vi "Configure Mask Test.vi"(0 "VISA resource name":refnum<visa-resource-name>, 1 "Enable Mask Test (T: Enable)":bool=TRUE, 5 "Mask Test Source (1: Channel 1)":i32(ring)=1 items=["Channel 1"=1, "Channel 2"=2, "Channel 3"=3, "Channel 4"=4, "Function 1"=5, "Function 2"=6, "Function 3"=7, "Function 4"=8, "Differential 1"=61, "Differential 2"=62, "Common 1"=71, "Common 2"=72, "Equalized"=18], 7 "Mask Trigger Source (1: Channel 1)":i32(ring)=1 items=["Channel 1"=1, "Channel 2"=2, "Channel 3"=3, "Channel 4"=4], 9 "Impedance (0: None)":i32(ring) items=["None", "IMP75", "IMP100", "IMP110", "IMP120"], 11 "error in (no error)":errorcluster, 12 "Run":T2={"Enable Stop on Fail (F: Disable)"=FALSE, "Run Mode (0: Forever)"=0, "Waveform Count (1000)"=1000, "Time (1.0 min)"=1.0} {"Time (1.0 min)" format="%#.1g"; "Run Mode (0: Forever)" items=["Forever", "Waveform", "Time"]}, 13 "Test Options":T3={"Enable Averaging (F: Disable)"=FALSE, "Average Count (16)"=16, "Enable Use File Setup (T: Enable)"=TRUE}, 14 "Pulse Amplitude":T1={"Maximum Amplitude (1 V)"=1.0, "Minimum Amplitude (1 V)"=1.0}) -> (4 "VISA resource name out":refnum<visa-resource-name>, 15 "error out":errorcluster)   [LabVIEW 2013, in "Agilent 90000 Series.lvlib"]
doc: "Configures the mask test and the parameters required for a mask test. This VI has to be called before calling any other mask related VIs."
uses:
  Agilent 90000 Series.lvlib
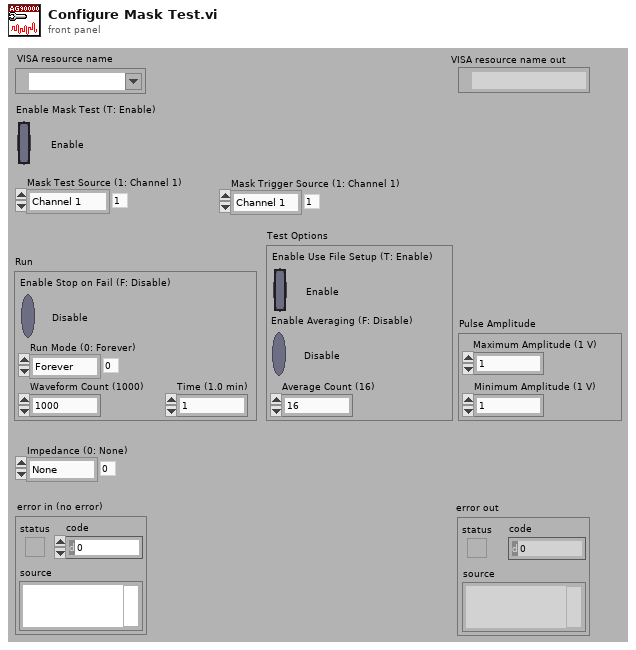
[diagram p1: front panel]
types:
  T1 = cluster{"Maximum Amplitude (1 V)":dbl, "Minimum Amplitude (1 V)":dbl}
  T2 = cluster{"Enable Stop on Fail (F: Disable)":bool, "Run Mode (0: Forever)":i32, "Waveform Count (1000)":i32, "Time (1.0 min)":dbl}
  T3 = cluster{"Enable Averaging (F: Disable)":bool, "Average Count (16)":i32, "Enable Use File Setup (T: Enable)":bool}
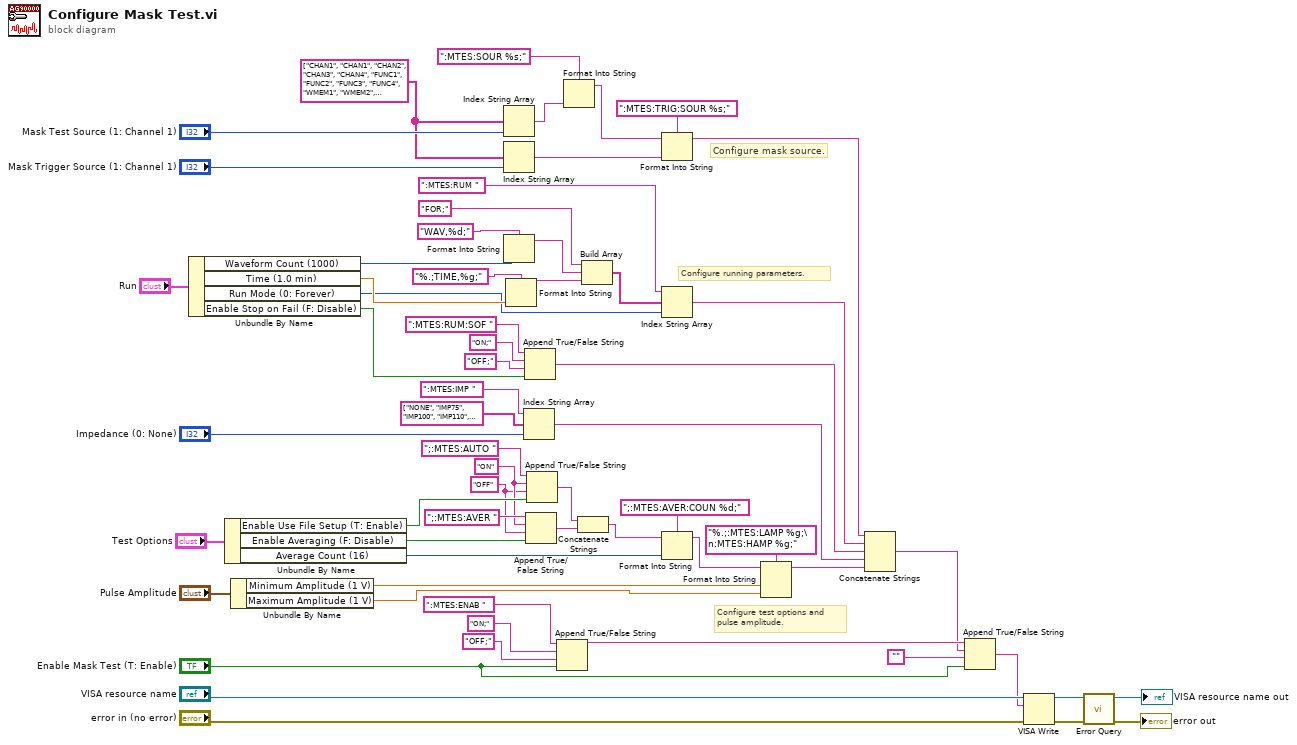
[diagram p0: block diagram]
diagram:
  w1 = string[] ["CHAN1", "CHAN1", "CHAN2", "CHAN3", "CHAN4", "FUNC1", "FUNC2", "FUNC3", "FUNC4", "WMEM1", "WMEM2", "WMEM3", "WMEM4", "AUX", "LINE", "CLOC", "MTR", "MSP", "EQU", "NONE", "DIG0", "DIG1", "DIG2", "DIG3", "DIG4", "DIG5", "DIG6", "DIG7", "DIG8", "DIG9", "DIG10", "DIG11", "DIG12", "DIG13", "DIG14", "DIG15", "", "", "", "", "", "POD1", "POD2", "", "", "", "", "", "", "", "", "BUS1", "BUS2", "BUS3", "BUS4", "", "", "", "", "", "", "DIFF1", "DIFF2", "", "", "", "", "", "", "", "", "COMM3", "COMM4"]
  w8 = "OFF" ("false string")
  w9 = "ON" ("true string")
  # "Configure running parameters."
  # "Configure test options and\npulse amplitude."
  # "Configure mask source."
  n1 = Unbundle By Name("Run") -> ("Waveform Count (1000)"=w49:i32, "Time (1.0 min)"=w47:dbl, "Run Mode (0: Forever)"=w41:i32, "Enable Stop on Fail (F: Disable)"=w39:bool)
  n2 = Unbundle By Name("Test Options") -> ("Enable Use File Setup (T: Enable)"=w13:bool, "Enable Averaging (F: Disable)"=w31:bool, "Average Count (16)"=w32:i32)
  n3 = Unbundle By Name("Pulse Amplitude") -> ("Minimum Amplitude (1 V)"=w29:dbl, "Maximum Amplitude (1 V)"=w28:dbl)
  n4 = Index String Array(1:"Mask Test Source (1: Channel 1)", 2:w1) -> (0:w53:string)  [unwired: 1 out]
  n5 = Index String Array(1:"Mask Trigger Source (1: Channel 1)", 2:w1) -> (0:w6:string)  [unwired: 1 out]
  n6 = Format Into String(format string="WAV,%d;", w49) -> (resulting string=w44:string)  [unwired: 2 in, 1 out]
  n7 = Format Into String(format string="%.;TIME,%g;", w47) -> (resulting string=w46:string)  [unwired: 2 in, 1 out]
  n8 = Index String Array(1:"Impedance (0: None)", 2:string[] ["NONE", "IMP75", "IMP100", "IMP110", "IMP120"] ("string array"), 3:":MTES:IMP " ("string (\"\")")) -> (0:w21:string)
  n9 = Append True/False String(1:w39, 2:"OFF;" ("false string"), 3:"ON;" ("true string"), 4:":MTES:RUM:SOF " ("string (\"\")")) -> (0:w4:string)
  n10 = Append True/False String(1:w31, 2:w8, 3:w9, 4:";:MTES:AVER " ("string (\"\")")) -> (0:w10:string)
  n11 = Append True/False String(1:w13, 2:w8, 3:w9, 4:";:MTES:AUTO " ("string (\"\")")) -> (0:w12:string)
  n12 = Append True/False String(1:"Enable Mask Test (T: Enable)", 2:"OFF;" ("false string"), 3:"ON;" ("true string"), 4:":MTES:ENAB " ("string (\"\")")) -> (0:w18:string)
  n13 = Format Into String(format string=":MTES:SOUR %s;", w53) -> (resulting string=w5:string)  [unwired: 2 in, 1 out]
  n14 = Concatenate Strings(w12, w10) -> (w11:string)
  n15 = Build Array("FOR;", w44, w46) -> (w42:string[])
  n16 = Format Into String(format string=":MTES:TRIG:SOUR %s;", initial string=w5, w6) -> (resulting string=w2:string)  [unwired: 1 in, 1 out]
  n17 = Index String Array(1:w41, 2:w42, 3:":MTES:RUM " ("string (\"\")")) -> (0:w3:string)
  n18 = Format Into String(format string=";:MTES:AVER:COUN %d;", initial string=w11, w32) -> (resulting string=w26:string)  [unwired: 1 in, 1 out]
  n19 = Format Into String(format string="%.;:MTES:LAMP %g;\n:MTES:HAMP %g;", initial string=w26, w29, w28) -> (resulting string=w25:string)  [unwired: 1 in, 1 out]
  n20 = Concatenate Strings(w2, w3, w4, w21, w25) -> (w17:string)
  n21 = Append True/False String(1:"Enable Mask Test (T: Enable)", 2:"", 3:w17, 4:w18) -> (0:w16:string)
  n22 = VISA Write(VISA resource name="VISA resource name", write buffer=w16, error in (no error)="error in (no error)") -> (VISA resource name out=w60:refnum<visa-resource-name>, error out=w59:errorcluster)  [unwired: 1 out]
  n23 = call "Error Query.vi"("error in (no error)"=w59, "VISA resource name"=w60) -> ("error out"=→"error out":errorcluster, "VISA resource name out"=→"VISA resource name out":refnum<visa-resource-name>)  [unwired: 8 out]
